vi "Read Message.vi"(8 "error in (no error)":errorcluster, 11 "RemoteControl in":refnum<class "RemoteControl.lvclass">) -> (0 "error out":errorcluster, 1 "Data":string, 2 "Command":string, 3 "RemoteControl out":refnum<class "RemoteControl.lvclass">, 4 "ID":string)   [LabVIEW 2019, in "RemoteControl.lvclass"]
uses:
  RemoteControl.lvclass
  RemoteControl.lvclass/RemoteControl.ctl
  Typedefs/Message--Cluster.ctl
  20f6ee6e-4e02-4e70-bcae-a5921812ef1c.vi
  Private/RemoteControl.GlobalVariable.vi
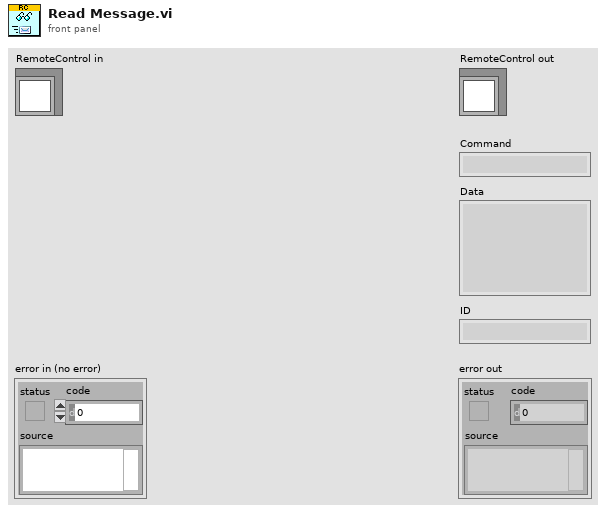
[diagram p1: front panel]
types:
  T1 = typedef "RemoteControl.lvclass/RC Process Type--Enum.ctl" = enum16{"Listener", "Server", "Client"}
  T2 = typedef "RemoteControl.lvclass/Message--Cluster.ctl" = cluster{"Command":string, "Data":variant, "ID":string}
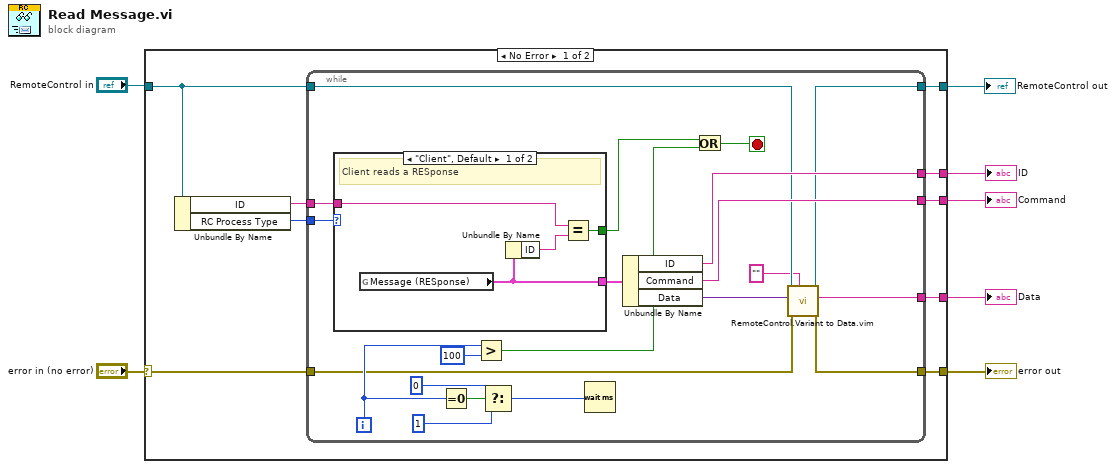
[diagram p0: block diagram]
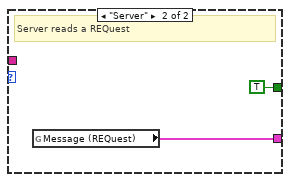
[diagram p2: hidden frame]
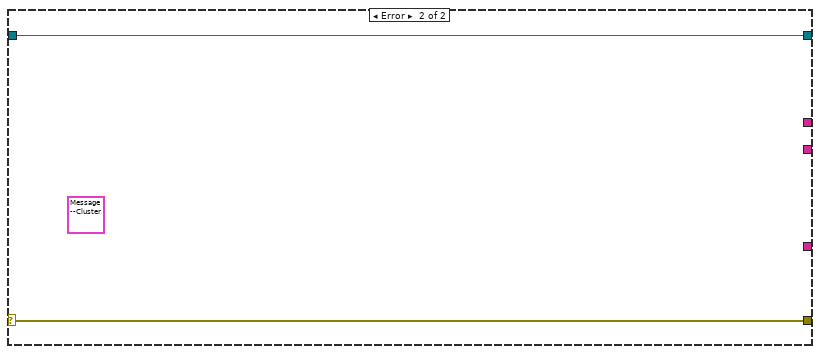
[diagram p3: hidden frame]
diagram:
  n1 = case shown="No Error" "error in (no error)" {
    selector: "error in (no error)" -> [w15 w44]
    tunnel: [w9 w45] -> w5
    tunnel: "RemoteControl in" -> [w8 w45]
    tunnel: [w16 _] -> w4
    tunnel: [w12 _] -> w3
    tunnel: [w11 _] -> w2
    tunnel: [w14 w44] -> w1
    frame No Error {
      n2 = Unbundle By Name(w8) -> ("ID"=w10:string, "RC Process Type"=w13:T1)
      n3 = while {
        tunnel: [w20] -> w16
        tunnel: w13 -> [w37]
        tunnel: [w34] -> w12
        tunnel: [w35] -> w11
        tunnel: w10 -> [w33]
        tunnel: w15 -> [w19]
        tunnel: [w18] -> w14
        tunnel: w8 -> [w23]
        tunnel: [w17] -> w9
        i -> [w28]
        stop <- w25 stop-if-true
        n4 = case shown="\"Client\", Default" w37 {
          tunnel: [w41 w43] -> w36
          tunnel: w33 -> [w38 _]
          tunnel: [w40 TRUE] -> w26
          frame "Client", Default {
            # "Client reads a RESponse"
            n5 = global read "RemoteControl.GlobalVariable.vi" "Message (RESponse)"() -> (w41:T2)
            n6 = Unbundle By Name(w41) -> ("ID"=w39:string)
            n7 = Equal?(x=w38, y=w39) -> (x = y?=w40:bool)
          }
          frame "Server" {
            # "Server reads a REQuest"
            n8 = global read "RemoteControl.GlobalVariable.vi" "Message (REQuest)"() -> (w43:T2)
          }
        }
        n9 = Equal To 0?(x=w28) -> (x = 0?=w32:bool)
        n10 = Greater?(x=w28, y=100) -> (0:w24:bool)
        n11 = Select(t=u32 0 ("milliseconds to wait"), s=w32, f=u32 1 ("milliseconds to wait")) -> (s? t:f=w29:u32)
        n12 = Wait (ms)(milliseconds to wait=w29) -> ()  [unwired: 1 out]
        n13 = Unbundle By Name(w36) -> ("ID"=w35:string, "Command"=w34:string, "Data"=w22:variant)
        n14 = Or(x=w26, y=w24) -> (x .or. y?=w25:bool)
        n15 = call "RemoteControl.Variant to Data.vim"("Data Type"="", "error in (no error)"=w19, "Data in"=w22, "RemoteControl in"=w23) -> ("error out"=w18:errorcluster, "Data out"=w20:string, "RemoteControl out"=w17:refnum<class "RemoteControl.lvclass">)  [unwired: 5 in]
      }
    }
    frame Error {
      (unwired) T2 {"Command"="", "Data"=variant(string ""), "ID"=""} ("Message")
    }
  }
  "error out" <- w1
  "RemoteControl out" <- w5
  "ID" <- w2
  "Command" <- w3
  "Data" <- w4
